vi "Execute PID Controllers.vi"(8 "error in (no error)":errorcluster, 11 "State Variables in":T1 {"Config"."Config"."Industrial Settings"."Write Refs"."Data Reference" format="%.0x"; "Config"."Config"."Industrial Settings"."Read Refs"."Data Reference" format="%.0x"; "Config"."Config"."PID Settings"."Read Refs"."Data Reference" format="%.0x"; "Config"."Config"."PID Settings"."Write Refs"."Data Reference" format="%.0x"}) -> (0 "error out":errorcluster, 3 "State Variables out":T1 {"Config"."Config"."Industrial Settings"."Write Refs"."Data Reference" format="%.0x"; "Config"."Config"."Industrial Settings"."Read Refs"."Data Reference" format="%.0x"; "Config"."Config"."PID Settings"."Read Refs"."Data Reference" format="%.0x"; "Config"."Config"."PID Settings"."Write Refs"."Data Reference" format="%.0x"})   [LabVIEW 2013, in "Control Addon Engine.lvlib"]
uses:
  Control Addon Engine.lvlib
  Types/RT Driver State Variables.ctl
  Types/RT Configuration.ctl
  Shared/Types/Gain Schedule.ctl
  Shared/Types/Compiled Settings.ctl
  Shared/Types/Compiled PID Settings.ctl
  <vilib>/NI Veristand/Custom Device API/Block Data Reference.ctl
  <vilib>/NI Veristand/Custom Device API/Data Reference.ctl
  Shared/Types/Compiled Industrial Settings.ctl
  Shared/Types/Compiled Industrial Parameters.ctl
  <vilib>/NI Veristand/Custom Device API/Custom Device Engine Event Ref.ctl
  <vilib>/addons/control/pid/pid.llb/PID Derivative Action Buffered (DBL Array).vi
  <vilib>/addons/control/pid/pid.llb/PID Get Advanced Error (DBL Array).vi
  <vilib>/addons/control/pid/pid.llb/PID Integral Action Buffered (DBL Array).vi
  <vilib>/addons/control/pid/pid.llb/PID Resize 1D Array.vi
  <vilib>/addons/control/pid/pid.llb/PID Get Advanced Error (DBL).vi
  <vilib>/addons/control/pid/pid.llb/PID Output Rate Limiter (DBL Array).vi
  <vilib>/NI Veristand/Custom Device API/Global Data Refs.vi
  <vilib>/addons/control/pid/pid.llb/PID Gain Schedule.vi
  <vilib>/addons/control/pid/pid.llb/PID Gain Schedule (DBL).vi
  <vilib>/addons/control/pid/pid.llb/PID Parameter Manager (DBL Array).vi
  <vilib>/NI Veristand/Custom Device API/Custom Device API.lvlib
  <vilib>/addons/control/pid/NI_PID_pid.lvlib
  Shared/Control Addon Shared.lvlib
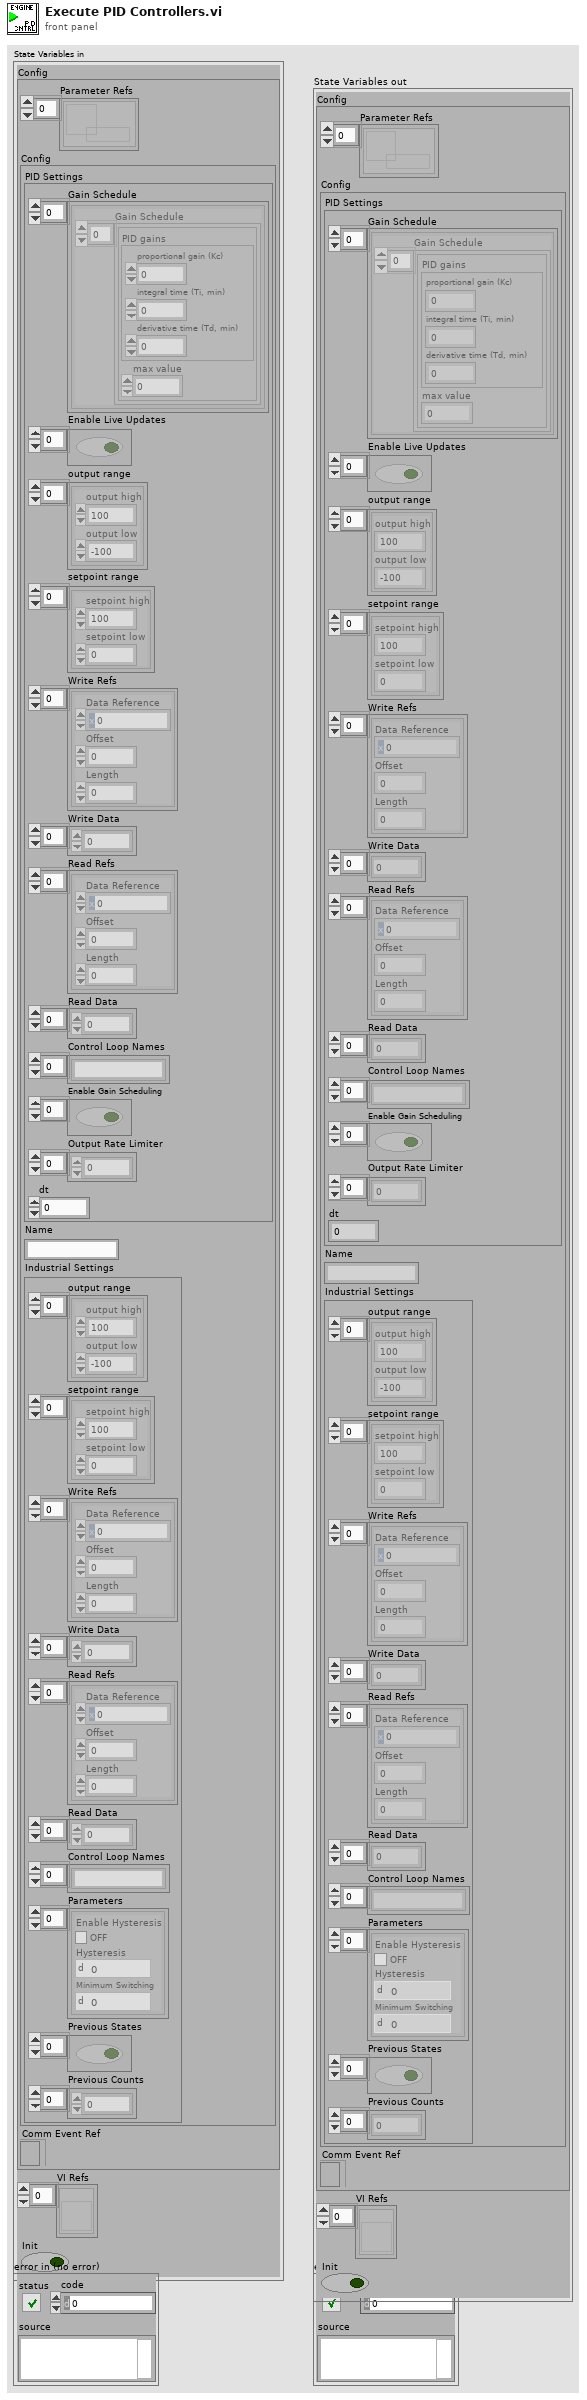
[diagram p1: front panel]
types:
  T1 = typedef "Control Addon Engine.lvlib/RT Driver State Variables.ctl" = cluster{"Config":T2, "VI Refs":refnum<vi>[], "Init":bool}
  T2 = typedef "Control Addon Engine.lvlib/RT Configuration.ctl" = cluster{"Parameter Refs":refnum<data-value>[], "Config":T3, "Comm Event Ref":T10}
  T3 = typedef "Control Addon Shared.lvlib/Compiled Settings.ctl" = cluster{"PID Settings":T4, "Name":string, "Industrial Settings":T8}
  T4 = typedef "Control Addon Shared.lvlib/Compiled PID Settings.ctl" = cluster{"Gain Schedule":T5[], "Enable Live Updates":bool[], "output range":cluster{"output high":dbl, "output low":dbl}[], "setpoint range":cluster{"setpoint high":dbl, "setpoint low":dbl}[], "Write Refs":T6[], "Write Data":dbl[], "Read Refs":T6[], "Read Data":dbl[], "Control Loop Names":string[], "Enable Gain Scheduling":bool[], "Output Rate Limiter":dbl[], "dt":dbl}
  T5 = typedef "Control Addon Shared.lvlib/Gain Schedule.ctl" = cluster{"Gain Schedule":cluster{"PID gains":cluster{"proportional gain (Kc)":dbl, "integral time (Ti, min)":dbl, "derivative time (Td, min)":dbl}, "max value":dbl}[]}
  T6 = typedef "Custom Device API.lvlib/Block Data Reference.ctl" = cluster{"Data Reference":T7, "Offset":i32, "Length":i32}
  T7 = typedef "Custom Device API.lvlib/Data Reference.ctl" = i32
  T8 = typedef "Control Addon Shared.lvlib/Compiled Industrial Settings.ctl" = cluster{"output range":cluster{"output high":dbl, "output low":dbl}[], "setpoint range":cluster{"setpoint high":dbl, "setpoint low":dbl}[], "Write Refs":T6[], "Write Data":dbl[], "Read Refs":T6[], "Read Data":dbl[], "Control Loop Names":string[], "Parameters":T9[], "Previous States":bool[], "Previous Counts":u64[]}
  T9 = typedef "Control Addon Shared.lvlib/Compiled Industrial Parameters.ctl" = cluster{"Enable Hysteresis":bool, "Hysteresis":dbl, "Minimum Switching":u64}
  T10 = typedef "Custom Device API.lvlib/Custom Device Engine Event Ref.ctl" = refnum<event-registration>
  T11 = cluster{"setpoint high":dbl, "setpoint low":dbl}[]
  T12 = cluster{"proportional gain (Kc)":dbl, "integral time (Ti, min)":dbl, "derivative time (Td, min)":dbl}[]
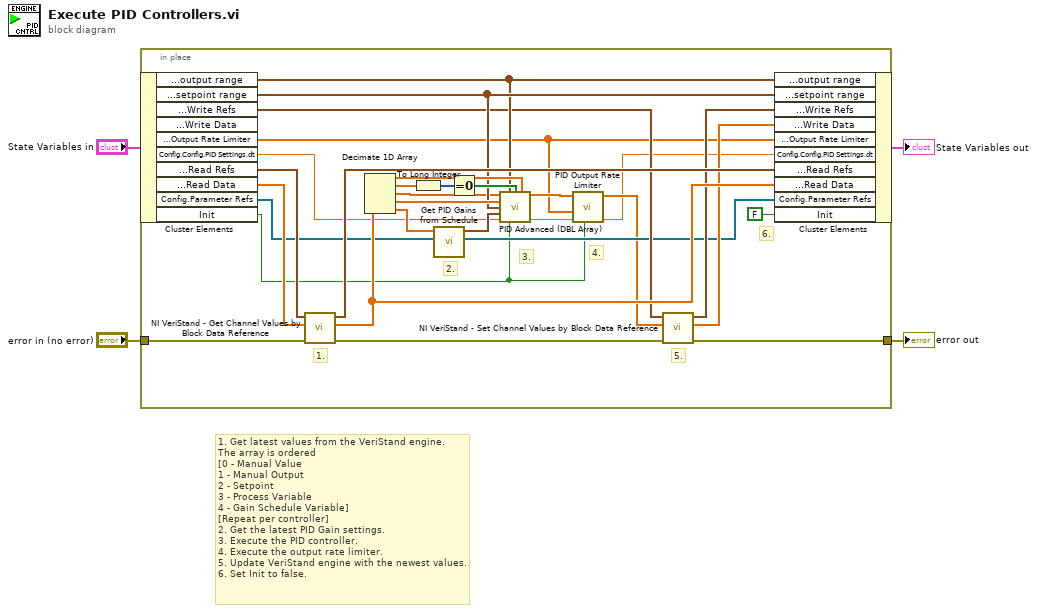
[diagram p0: block diagram]
diagram:
  # "1. Get latest values from the VeriStand engine.\nThe array is ordered\n[0 - Manual Value\n1 - Manual Output\n2 - Setpoint\n3 - Process Variable\n4 - Gain Schedule Variable]\n[Repeat per controller]\n2. Get the latest PID Gain settings.\n3. Execute the PID controller.\n4. Execute the output rate limiter.\n5. Update VeriStand engine with the newest values.\n6. Set Init to false."
  n1 = in-place {
    in-place-border: "error in (no error)" -> [w34]
    in-place-border: [w20] -> w4
    # "6."
    # "5."
    # "4."
    # "3."
    # "2."
    # "1."
    n2 = in-place-cluster #1("State Variables in") -> ("Config.Config.PID Settings.output range"=w21:cluster{"output high":dbl, "output low":dbl}[], "Config.Config.PID Settings.setpoint range"=w22:T11, "Config.Config.PID Settings.Write Refs"=w19:T6[], "Config.Config.PID Settings.Output Rate Limiter"=w10:dbl[], "Config.Config.PID Settings.dt"=w8:dbl, "Config.Config.PID Settings.Read Refs"=w33:T6[], "Config.Config.PID Settings.Read Data"=w32:dbl[], "Config.Parameter Refs"=w15:refnum<data-value>[], "Init"=w6:bool)  [unwired: 1 out]
    n3 = call <vilib>:"NI VeriStand - Get Channel Values by Block Data Reference.vi"("error in (no error)"=w34, "Values Array in"=w32, "Block Data Ref"=w33) -> ("error out"=w29:errorcluster, "Values Array out"=w28:dbl[], "Block Data Ref dup"=w30:T6[])  [unwired: 6 in]
    n4 = Decimate 1D Array(w28) -> (w27:dbl[], w25:dbl[], w13:dbl[], w24:dbl[], w16:dbl[])
    n5 = To Long Integer(number=w25) -> (32bit integer=w31:i32[])
    n6 = call "Get PID Gains from Schedule.vi"("Parameter Refs"=w15, "Gain Schedule Value"=w16) -> ("Parameter Refs"=w14:refnum<data-value>[], "PID"=w23:T12)  [unwired: 8 in]
    n7 = Equal To 0?(x=w31) -> (x = 0?=w26:bool[])
    n8 = call <vilib>:"PID Advanced (DBL Array).vi"("setpoint"=w13, "output range"=w21, "auto? (T)"=w26, "manual control"=w27, "process variable"=w24, "setpoint range"=w22, "PID gains"=w23, "dt (s)"=w8, "reinitialize? (F)"=w6) -> ("output"=w12:dbl[], "dt out (s)"=w9:dbl)  [unwired: 5 in]
    n9 = call-poly <vilib>:"PID Output Rate Limiter.vi"("reinitialize? (F)"=w6, "dt (s)"=w9, "output rate (EGU/min)"=w10, "input (controller output)"=w12) -> ("dt out (s)"=w7:dbl, "output"=w11:dbl[])  [unwired: 4 in]
    n10 = call <vilib>:"NI VeriStand - Set Channel Values by Block Data Reference.vi"("error in (no error)"=w29, "Values Array in"=w11, "Block Data Ref"=w19) -> ("error out"=w20:errorcluster, "Values Array out"=w18:dbl[], "Block Data Ref dup"=w17:T6[])  [unwired: 6 in]
    n11 = in-place-cluster #1("Config.Config.PID Settings.output range"=w21, "Config.Config.PID Settings.setpoint range"=w22, "Config.Config.PID Settings.Write Refs"=w17, "Config.Config.PID Settings.Write Data"=w18, "Config.Config.PID Settings.Output Rate Limiter"=w10, "Config.Config.PID Settings.dt"=w7, "Config.Config.PID Settings.Read Refs"=w30, "Config.Config.PID Settings.Read Data"=w28, "Config.Parameter Refs"=w14, "Init"=FALSE) -> (→"State Variables out":T1)
  }
  "error out" <- w4
